vi "Read Hardware.vi"(11 "DAC in":refnum<class "DAC.lvclass">) -> (2 "Hardware.lvlib:Hardware.lvclass":refnum<class "Hardware.lvclass">, 3 "DAC out":refnum<class "DAC.lvclass">)   [LabVIEW 2019]
uses:
  DAC.lvclass
  Hardware/Hardware.lvclass
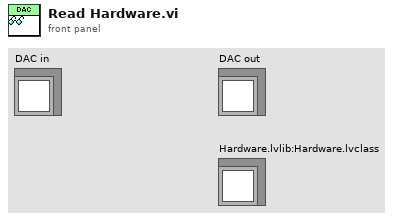
[diagram p1: front panel]
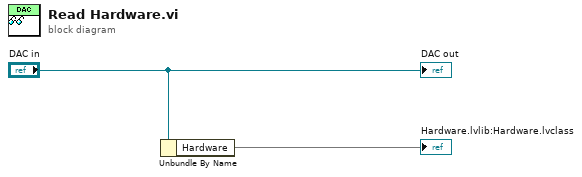
[diagram p0: block diagram]
diagram:
  n1 = Unbundle By Name("DAC in") -> ("Hardware"=→"Hardware.lvlib:Hardware.lvclass")
  "DAC out" <- "DAC in"
